vi "Delay.vi"(11 "error in":errorcluster, 13 "delay (1 sec)":dbl=1.0) -> (15 "error out":errorcluster)   [LabVIEW 2015, in "_Unit Tests Shared.lvlib"]
uses:
  _Unit Tests Shared.lvlib
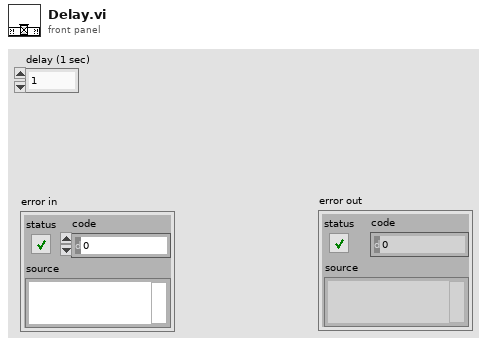
[diagram p1: front panel]
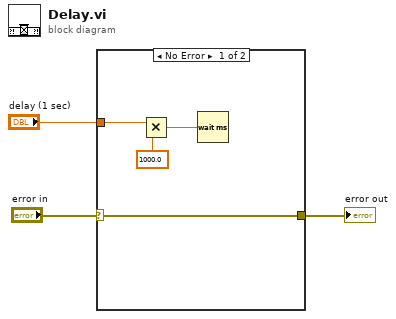
[diagram p0: block diagram]
diagram:
  n1 = case shown="No Error" "error in" {
    selector: "error in" -> [w6 w8]
    tunnel: [w6 w8] -> w2
    tunnel: "delay (1 sec)" -> [w7 _]
    frame No Error {
      n2 = Multiply(x=w7, y=1000.0) -> (x*y=w4:dbl)
      n3 = Wait (ms)(milliseconds to wait=w4) -> ()  [unwired: 1 out]
    }
    frame Error {
    }
  }
  "error out" <- w2
